vi "Subscribe.vi"(8 "error in (no error)":errorcluster, 10 "SubscriptionRequest":refnum<class "SubscriptionRequest.lvclass">, 11 "IObserver in":refnum<class "IObserver.lvclass">) -> (0 "error out":errorcluster, 3 "IObserver out":refnum<class "IObserver.lvclass">)   [LabVIEW 2017, in "IObserver.lvlib" / "IObserver.lvclass"]
doc: "<License>\nCopyright © 2017 Composed Systems, LLC | All rights reserved\nwww.composed.io\n\nAuthor: Ethan Stern <ethan.stern@composed.io>\n\nThis software is provided \"AS IS\" WITHOUT WARRANTIES, either express or implied, AND IS FOR EDUCATIONAL PURPOSES ONLY.\n</License>"
uses:
  <vilib>/gpm_packages/@cs/mva-core/Source/IObserver/IObserver/IObserver.lvclass
  <vilib>/gpm_packages/@cs/mva-core/Source/IMediator/SubscriptionRequest/SubscriptionRequest.lvclass
  <vilib>/gpm_packages/@cs/mva-core/Source/IObserver/IObserver/IObserver.lvclass/IObserver.ctl
  <vilib>/gpm_packages/@cs/mva-core/Source/IMediator/IMediator Messages/Subscribe Msg/Subscribe Msg.lvclass/Subscribe Msg.ctl
  <vilib>/gpm_packages/@cs/actor-framework-messages/Source/RoundTripMessage/RoundTripMessage.lvclass/RoundTripMessage.ctl
  <vilib>/ActorFramework/Message Enqueuer/Message Enqueuer.lvclass/Message Enqueuer.ctl
  <vilib>/gpm_packages/@cs/actor-framework-messages/Source/RoundTripMessage/Return Round-Trip Message.vi
  <vilib>/ActorFramework/Message Enqueuer/Enqueue.vi
  <vilib>/gpm_packages/@cs/mva-core/Source/IMediator/IMediator Messages/Subscribe Msg/Subscribe Msg.lvclass
  C:/Program Files/National Instruments/LabVIEW 2017/vi.lib/gpm_packages/@cs/actor-framework-messages/Source/RoundTripMessage/RoundTripMessage.lvclass
  <vilib>/gpm_packages/@cs/actor-framework-messages/Source/RoundTripMessage/RoundTripMessage.lvclass
  C:/Program Files/National Instruments/LabVIEW 2017/vi.lib/ActorFramework/Message/Message.lvclass
  <vilib>/ActorFramework/Message Priority Queue/Priority Enqueue.vi
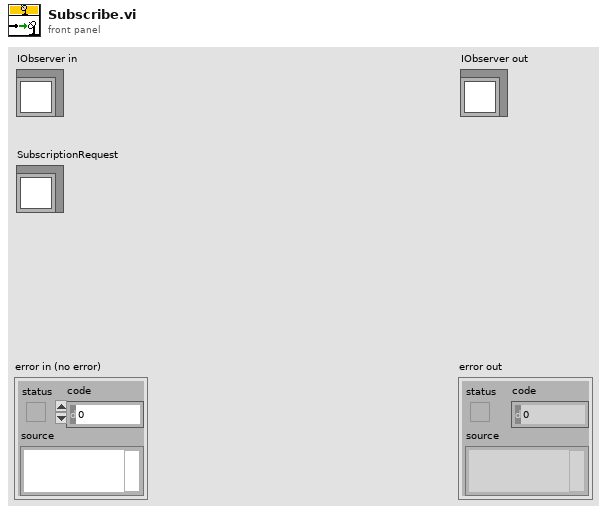
[diagram p1: front panel]
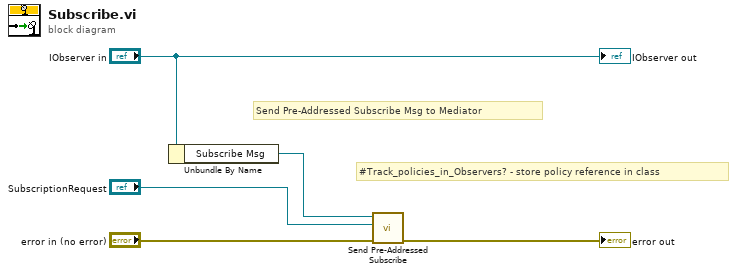
[diagram p0: block diagram]
diagram:
  # "#Track_policies_in_Observers? - store policy reference in class"
  # "Send Pre-Addressed Subscribe Msg to Mediator"
  n1 = Unbundle By Name("IObserver in") -> ("Subscribe Msg"=w4:refnum<class "Subscribe Msg.lvclass">)
  n2 = call <vilib>:"Send Pre-Addressed Subscribe.vi"("error in (no error)"="error in (no error)", "Subscription Request"="SubscriptionRequest", "Subscribe Msg"=w4) -> ("error out"=→"error out":errorcluster)  [unwired: 8 in]
  "IObserver out" <- "IObserver in"
